vi "UtilityLib.set color of GUI object.vi"(2 "GUI object Ref":refnum<vi>, 3 "valueStatus":T1, 4 "Blinking? (false)":bool, 5 "error in (no error)":errorcluster) -> (19 "error out":errorcluster)   [LabVIEW 2014, in "UtilityLib.lvlib"]
doc: "This VI sets the color of the label and and the caption of a GUI object which's reference is connected. In case of a valid reference the color is set depending on the \"state\" (see \"Sixcolor.vi\"). Optional the GUI object can be set to blink."
uses:
  UtilityLib.lvlib
  UtilityLib.valueStatus.ctl
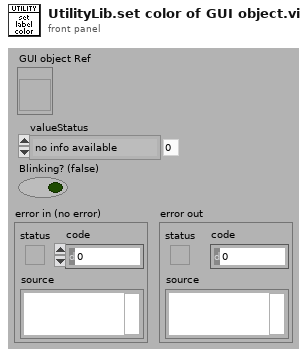
[diagram p1: front panel]
types:
  T1 = typedef "UtilityLib.lvlib/UtilityLib.valueStatus.ctl" = enum16{"no info available", "stand by/off", "on", "warning", "alarm/malfunction", "not implemented", "user action required", "important information", "system default", "control default", "indicator default", "button default"}
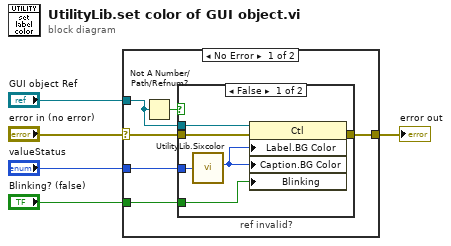
[diagram p0: block diagram]
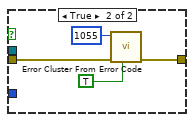
[diagram p2: hidden frame]
diagram:
  n1 = case shown="No Error" "error in (no error)" {
    selector: "error in (no error)" -> [w6 w22]
    tunnel: [w11 w22] -> w5
    tunnel: "GUI object Ref" -> [w10 _]
    tunnel: "Blinking? (false)" -> [w8 _]
    tunnel: "valueStatus" -> [w7 _]
    frame No Error {
      n2 = Not A Number/Path/Refnum?(number/path/refnum=w10) -> (NaN/Path/Refnum?=w9:bool)
      n3 = case "ref invalid?" shown="False" w9 {
        tunnel: w10 -> [w17 _]
        tunnel: w6 -> [w16 w21]
        tunnel: [w15 w20] -> w11
        tunnel: w7 -> [w14 _]
        tunnel: w8 -> [w13 _]
        frame False {
          n4 = call "UtilityLib.Sixcolor.vi"("State"=w14) -> ("elementBackground"=w12:u32)  [unwired: 2 in, 3 out]
          n5 = property class="Ctl"(reference=w17, error in=w16, "Label.BG Color"=w12, "Caption.BG Color"=w12, "Blinking"=w13) -> (error out=w15:errorcluster)  [unwired: 1 out]
        }
        frame True {
          n6 = call <vilib>:"Error Cluster From Error Code.vi"("show call chain? (False)"=TRUE, "error in (no error)"=w21, "error code (0)"=1055) -> ("error out"=w20:errorcluster)  [unwired: 6 in]
        }
      }
    }
    frame Error {
    }
  }
  "error out" <- w5
